vi "Number of Address Map Elements.vi"(2 "Configuration":refnum<class "AddressSpace.lvclass">) -> (6 "number of elements":u8)   [LabVIEW 2015, in "ScaleAndLimit.lvlib" / "AddressSpace.lvclass"]
uses:
  AddressSpace.lvclass
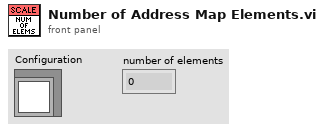
[diagram p1: front panel]
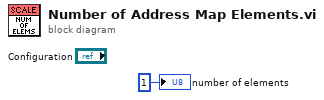
[diagram p0: block diagram]
diagram:
  "number of elements" <- u8 1 ("number of elements")
